vi "sv_Check for Frequency Change [Fract Octave].vi"(7 "reset filter (F)":bool, 8 "error in (no error)":errorcluster, 9 "frequency range [Hz]":T1={"low frequency"=125.0, "high frequency"=8000.0} {"high frequency" min=0.001 format="%.2f"; "low frequency" min=0.001 format="%.2f"}) -> (0 "error out":errorcluster, 2 "Param_has_changed":bool)   [LabVIEW 2017, in "SoundVib_Octave_2014 standard.lvlib"]
uses:
  <vilib>/addons/Sound and Vibration/svt_Octave/SoundVib_Octave_2014 standard.lvlib
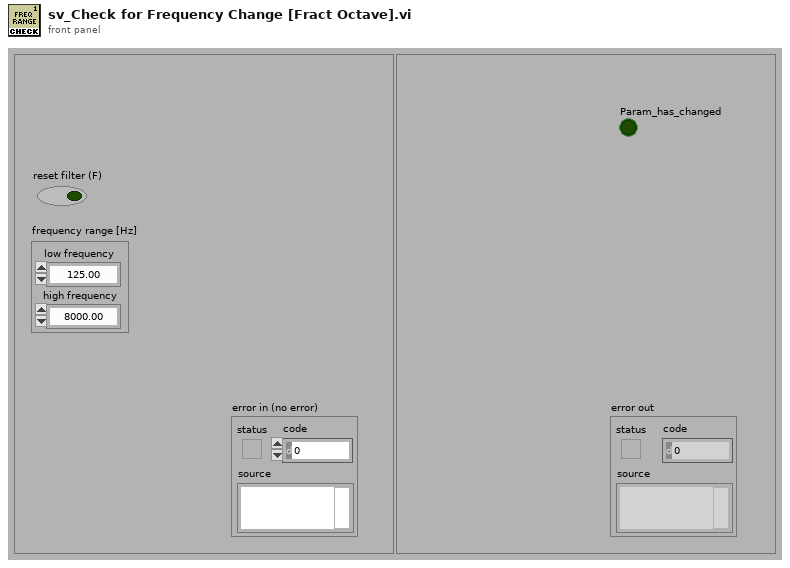
[diagram p1: front panel]
types:
  T1 = cluster{"low frequency":dbl, "high frequency":dbl}
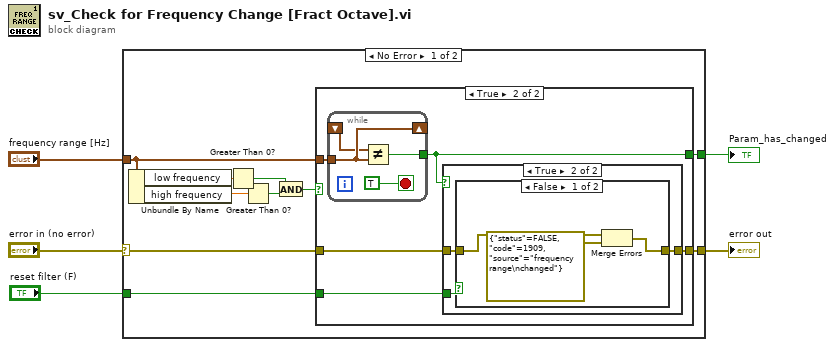
[diagram p0: block diagram]
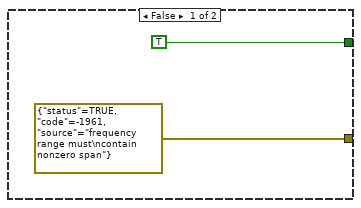
[diagram p2: hidden frame]
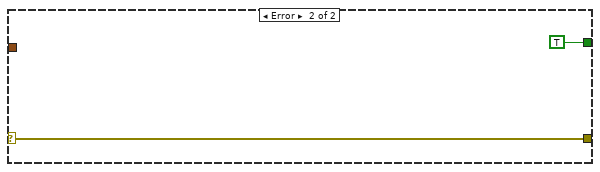
[diagram p5: hidden frame]
diagram:
  n1 = case shown="No Error" "error in (no error)" {
    selector: "error in (no error)" -> [w14 w36]
    tunnel: "frequency range [Hz]" -> [w12 _]
    tunnel: [w15 TRUE] -> w4
    tunnel: [w13 w36] -> w2
    tunnel: "reset filter (F)" -> [w6 _]
    frame No Error {
      n2 = Unbundle By Name(w12) -> ("low frequency"=w11:dbl, "high frequency"=w10:dbl)
      n3 = Greater Than 0?(x=w11) -> (x > 0?=w8:bool)
      n4 = Greater Than 0?(x=w10) -> (x > 0?=w9:bool)
      n5 = And(x=w8, y=w9) -> (x .and. y?=w7:bool)
      n6 = case shown="True" w7 {
        tunnel: [TRUE w22] -> w15
        tunnel: w14 -> [_ w21]
        tunnel: [errorcluster {"status"=TRUE, "code"=-1961, "source"="frequency range must\ncontain nonzero span"} ("error IO") w20] -> w13
        tunnel: w12 -> [_ w19]
        tunnel: w6 -> [_ w18]
        frame False {
        }
        frame True {
          n7 = while {
            tunnel: w19 -> [w24]
            tunnel: [w25] -> w22
            shift-left: _ -> [w23]
            shift-right: [w24] -> _
            stop <- TRUE stop-if-true
            n8 = Not Equal?(x=w23, y=w24) -> (x != y?=w25:bool)
          }
          n9 = case shown="True" w22 {
            tunnel: w21 -> [w27 w28]
            tunnel: [w27 w30] -> w20
            tunnel: w18 -> [_ w29]
            frame False {
            }
            frame True {
              n10 = case shown="False" w29 {
                tunnel: [w31 w34] -> w30
                tunnel: w28 -> [w33 w34]
                frame False {
                  n11 = Merge Errors(w33, errorcluster {"status"=FALSE, "code"=1909, "source"="frequency range\nchanged"} ("error IO")) -> (w31:errorcluster)
                }
                frame True {
                }
              }
            }
          }
        }
      }
    }
    frame Error {
    }
  }
  "error out" <- w2
  "Param_has_changed" <- w4
